vi "play formula.vi"() -> ()   [LabVIEW 2009]
uses:
  <vilib>/sound/lvsound.llb/Sound Format.ctl
  <vilib>/measure/NI_MABase.lvlib
  <vilib>/measure/NI_MAPro.lvlib
panel:
  in  "points":i32(slide) scale=4.0..44.0
  in  "Array":u8[](array[slide]) scale=0.0..100.0
  in  "square wave duty cycle (%)":dbl=50.0 format="%0.2f"
  in  "signal type":T1(ring)
  in  "sampling info":cluster{"Fs":dbl, "#s":dbl}={"Fs"=1000.0, "#s"=1000.0} {"Fs" format="%.2p"}
  in  "wait":u32
  in  "frequency":dbl(slide)=10.0 scale=10.0..30.0
  in  "formula":string="sin(w*t)*sin(2*pi(1)*t)"
  in  "stop":bool
  in  "player controls":cluster{"play/pause":bool, "volume":dbl}={"play/pause"=FALSE, "volume"=1.0} {"volume" scale=0.0037..1.0}
  out "Waveform graph":waveform(i16)(graph)
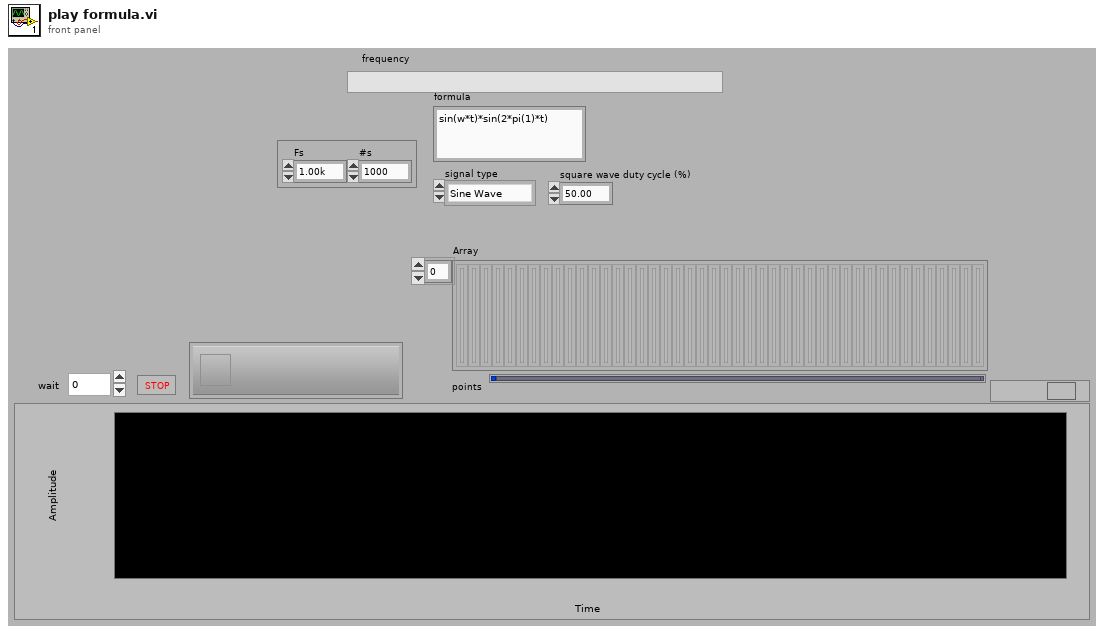
[diagram p1: front panel]
types:
  T1 = enum16{"Sine Wave", "Triangle Wave", "Square Wave", "Sawtooth Wave"}
  T2 = typedef "Sound Format.ctl" = cluster{"sound quality":enum16{"mono", "stereo"}, "rate":enum16{"11025", "22050", "44100", "8000"}, "bits per sample":enum16{"8 bit", "16 bit"}}
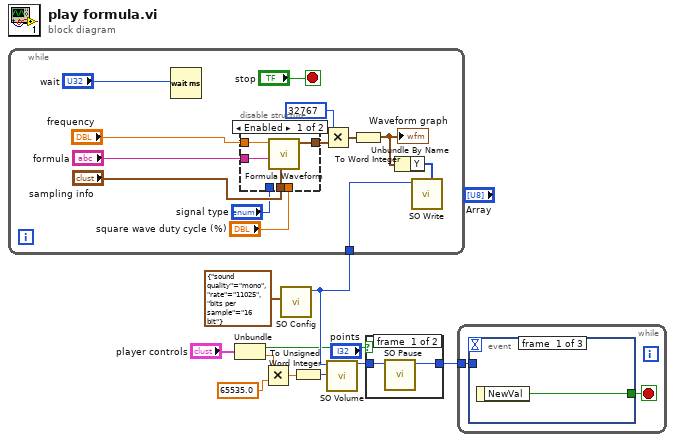
[diagram p0: block diagram]
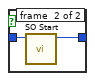
[diagram p2: hidden frame]
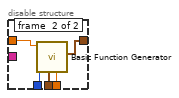
[diagram p3: hidden frame]
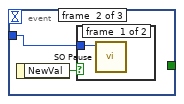
[diagram p4: hidden frame]
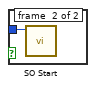
[diagram p5: hidden frame]
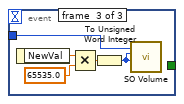
[diagram p6: hidden frame]
diagram:
  n1 = Unbundle("player controls") -> ("play/pause"=w3:bool, "volume"=w2:dbl)
  n2 = Multiply(x=w2, y=65535.0 ("left channel")) -> (x*y=w5:dbl)
  n3 = call <vilib>:"SO Config.vi"("sound format"=T2 {"sound quality"=enum."mono", "rate"=enum."11025", "bits per sample"=enum."16 bit"}) -> ("task ID out"=w8:u32)  [unwired: 9 in, 1 out]
  n4 = while {
    tunnel: w8 -> [w20]
    stop <- "stop" stop-if-true
    n5 = Wait (ms)(milliseconds to wait="wait") -> ()  [unwired: 1 out]
    n6 = disable-structure shown="Enabled" {
      disable-tunnel: "formula" -> [w27 _]
      disable-tunnel: "frequency" -> [w26 w31]
      disable-tunnel: [w25 w32] -> w19
      disable-tunnel: "sampling info" -> [w24 w30]
      disable-tunnel: "signal type" -> [_ w29]
      disable-tunnel: "square wave duty cycle (%)" -> [_ w28]
      frame #0 {
        n7 = call <vilib>:"Formula Waveform.vi"("sampling info"=w24, "formula"=w27, "frequency"=w26) -> ("signal out"=w25:waveform(dbl))  [unwired: 7 in, 1 out]
      }
      frame #1 {
        n8 = call <vilib>:"Basic Function Generator.vi"("square wave duty cycle (%)"=w28, "sampling info"=w30, "signal type"=w29, "frequency"=w31) -> ("signal out"=w32:waveform(dbl))  [unwired: 5 in, 2 out]
      }
    }
    n9 = Multiply(x=i16 32767, y=w19) -> (x*y=w13:waveform(dbl))
    n10 = To Word Integer(number=w13) -> (16bit integer=w12:waveform(i16))
    "Waveform graph" <- w12
    n11 = Unbundle By Name(w12) -> ("Y"=w14:i16[])
    n12 = call <vilib>:"SO Write.vi"("mono 16-bit"=w14, "task ID in"=w20) -> ()  [unwired: 8 in, 2 out]
  }
  n13 = To Unsigned Word Integer(number=w5) -> (unsigned 16bit integer=w6:u16)
  n14 = call <vilib>:"SO Volume.vi"("left channel"=w6, "task ID in"=w8) -> ("task ID out"=w9:u32)  [unwired: 8 in, 1 out]
  n15 = case shown="True" w3 {
    tunnel: w9 -> [w34 w36]
    tunnel: [w33 w35] -> w1
    frame #0 {
      n16 = call <vilib>:"SO Pause.vi"("task ID in"=w34) -> ("task ID out"=w33:u32)  [unwired: 9 in, 1 out]
    }
    frame #1 {
      n17 = call <vilib>:"SO Start.vi"("task ID in"=w36) -> ("task ID out"=w35:u32)  [unwired: 9 in, 1 out]
    }
  }
  n18 = while {
    tunnel: w1 -> [w37]
    stop <- w38 stop-if-true
    n19 = event shown="[1] \"player controls.play/pause\": Value Change" {
      selector: _ -> [_ _ _]
      dyn-events: _ -> [_ _ _]
      timeout: _ -> [_ _ _]
      tunnel: [w39 _ _] -> w38
      tunnel: w37 -> [_ w40 w44]
      event #0 {
        n20 = event-data() -> ("NewVal"=w39:bool)  [unwired: 1 in]
      }
      event #1 {
        n21 = event-data() -> ("NewVal"=w41:bool)  [unwired: 1 in]
        n22 = case shown="True" w41 {
          tunnel: w40 -> [w42 w43]
          frame #0 {
            n23 = call <vilib>:"SO Pause.vi"("task ID in"=w42) -> ()  [unwired: 9 in, 2 out]
          }
          frame #1 {
            n24 = call <vilib>:"SO Start.vi"("task ID in"=w43) -> ()  [unwired: 9 in, 2 out]
          }
        }
      }
      event #2 {
        n25 = event-data() -> ("NewVal"=w48:dbl)  [unwired: 1 in]
        n26 = Multiply(x=w48, y=65535.0 ("left channel")) -> (x*y=w46:dbl)
        n27 = To Unsigned Word Integer(number=w46) -> (unsigned 16bit integer=w47:u16)
        n28 = call <vilib>:"SO Volume.vi"("right channel"=w47, "left channel"=w47, "task ID in"=w44) -> ()  [unwired: 7 in, 2 out]
      }
    }
  }
